vi "Set Switches.vi"(8 "error in (no error)":errorcluster, 10 "switch states":bool[](array[boolean])=[FALSE, FALSE, FALSE, FALSE, FALSE, FALSE, FALSE, FALSE, FALSE, FALSE, FALSE, FALSE, FALSE, FALSE, FALSE, FALSE, FALSE, FALSE, FALSE, FALSE, FALSE, FALSE, FALSE, FALSE, FALSE, FALSE, FALSE, FALSE, FALSE, FALSE, FALSE, FALSE], 11 "MC switch refnum in":refnum<k24>) -> (0 "error out":errorcluster, 3 "MC switch refnum out":refnum<k24>)   [LabVIEW 2019, in "Minicircuit RF Switch Box.lvlib"]
doc: "Simultaneously sets all SPDT or transfer switches in a switch matrix. \n\n<b>switch states:</b> the array of the switch state. The sate of A is at the index 0 and H at the index 7."
uses:
  <instrlib>/Minicircuit RF Switch Box/Minicircuit RF Switch Box.lvlib
  C:/Program Files (x86)/National Instruments/LabVIEW 2019/instr.lib/Minicircuit RF Switch Box/mcl_RF_Switch_Controller_NET45.dll
  mcl_RF_Switch_Controller_NET45.dll
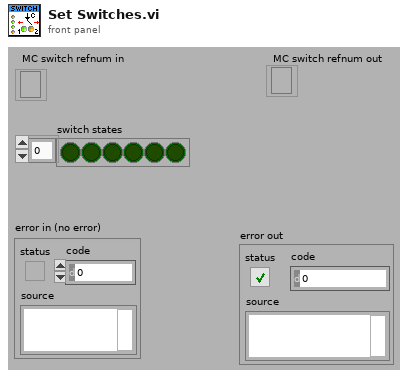
[diagram p1: front panel]
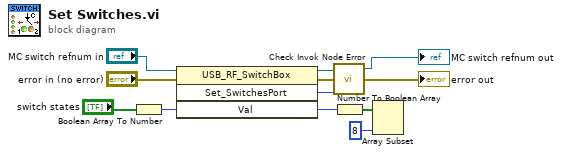
[diagram p0: block diagram]
diagram:
  n1 = Boolean Array To Number(Boolean array="switch states") -> (number=w1:u32)
  n2 = invoke class="USB_RF_SwitchBox" method="Set_SwitchesPort"(reference="MC switch refnum in", error in="error in (no error)", "Val"=w1) -> (reference out=w10:refnum<k24>, error out=w9:errorcluster, "Set_SwitchesPort"=w8:i32, "Val"=w5:u8)  [unwired: 1 in]
  n3 = call <instrlib>:"Check Invok Node Error.vi"("Connect"=w8, "error in (no error)"=w9, "MC switch refnum in"=w10) -> ("error out"=→"error out":errorcluster, "MC switch refnum out"=→"MC switch refnum out":refnum<k24>)  [unwired: 1 in]
  n4 = Number To Boolean Array(number=w5) -> (Boolean array=w4:bool[])
  n5 = Array Subset(array=w4, length=8) -> ()  [unwired: 1 in, 1 out]
